vi "Auton Abort.vi"(8 "error in":errorcluster) -> (0 "error out":errorcluster)   [LabVIEW 2016, in "Auton Mode Base.lvclass"]
uses:
  Auton Mode Base.lvclass
  Private/Auton Abort Global.vi
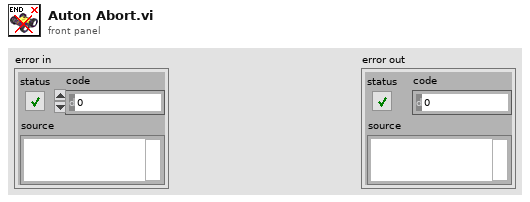
[diagram p1: front panel]
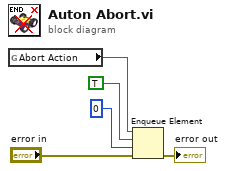
[diagram p0: block diagram]
diagram:
  n1 = global read "Auton Abort Global.vi" "Abort Action"() -> (w5:refnum<queue>)
  n2 = Enqueue Element(queue=w5, element=TRUE, timeout in ms (-1)=0, error in (no error)="error in") -> (error out=→"error out":errorcluster)  [unwired: 2 out]
